vi "固定站CODMn测量流程.vi"(11 "控制命令":T1(ring)) -> ()   [LabVIEW 2016, in "斯坦道CODMn.lvlib"]
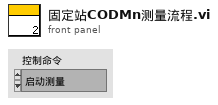
[diagram p1: front panel]
types:
  T1 = enum16{"启动测量", "标样核查", "零点核查", "跨度核查", "空白测试", "平行样测试", "加标回收", "空白校准", "标样校准", "初始化（清洗）", "停止测试", "仪器重启", "校时", "模式设置", "测量间隔设置"}
  T2 = cluster{"命令":string, "测量模式":enum16{"水样测量", "标样核查", "零点核查", "跨度核查", "空白测试", "加标回收", "平行样", "校零", "校标"}, "CODMn量程切换":enum32{"H", "L", "AUTO"}}
  T3 = cluster{"仪器":enum16{"", "氨氮", "总磷", "总氮", "CODMn", "CODCr"}, "启动命令":enum16{"启动水样流程", "启动加标流程", "排液", "停止", "柱塞泵启动"}}
  T4 = cluster{"时间标识":timestamp, "参数":string, "日志信息":string, "流程参数":string}
  T5 = enum16{"水样测量", "标样核查", "零点核查", "跨度核查", "空白测试", "加标回收", "平行样", "校零", "校标"}
  T6 = cluster{"时间标识":timestamp, "设备":string, "日志信息":string, "流程参数":string}
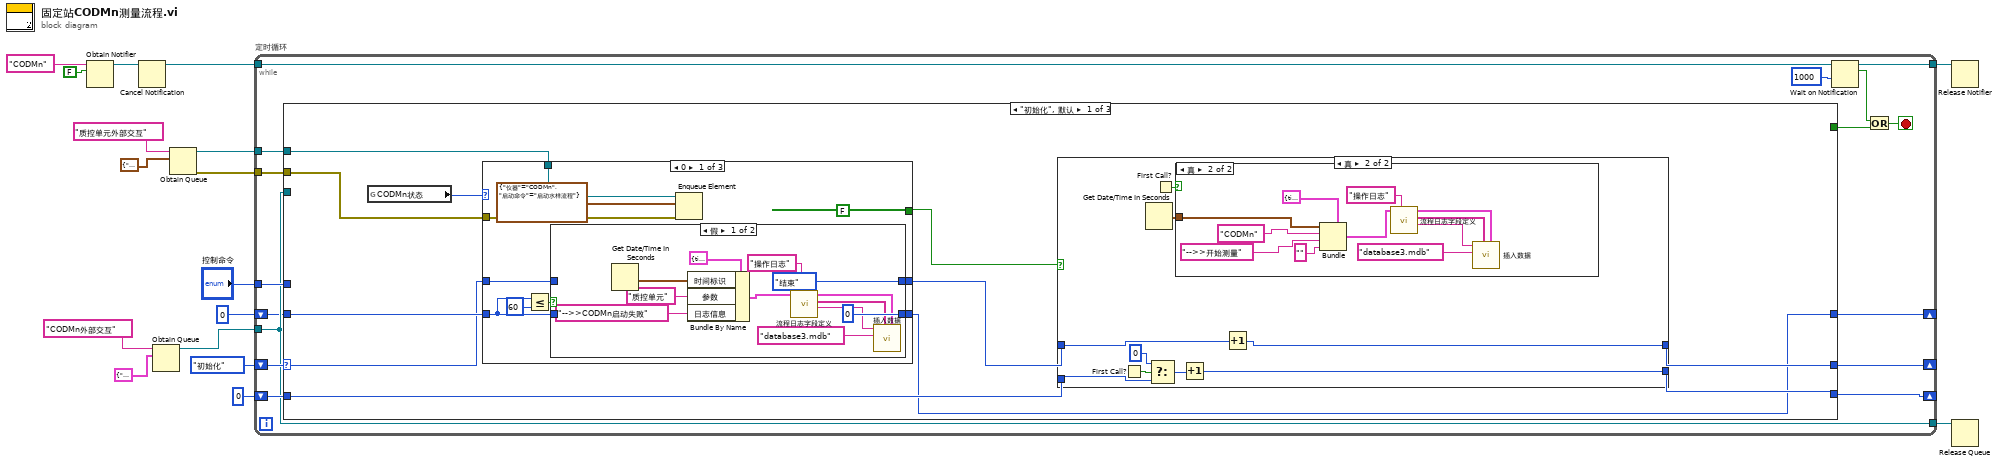
[diagram p0: block diagram]
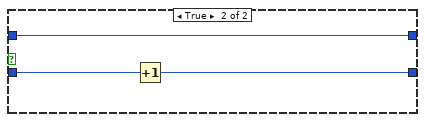
[diagram p4: hidden frame]
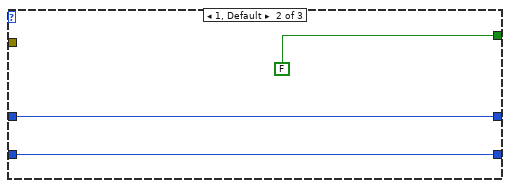
[diagram p5: hidden frame]
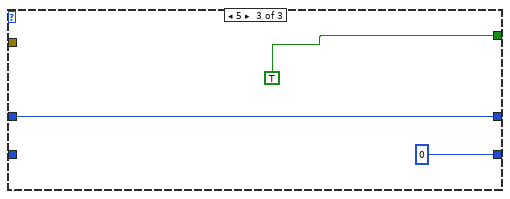
[diagram p6: hidden frame]
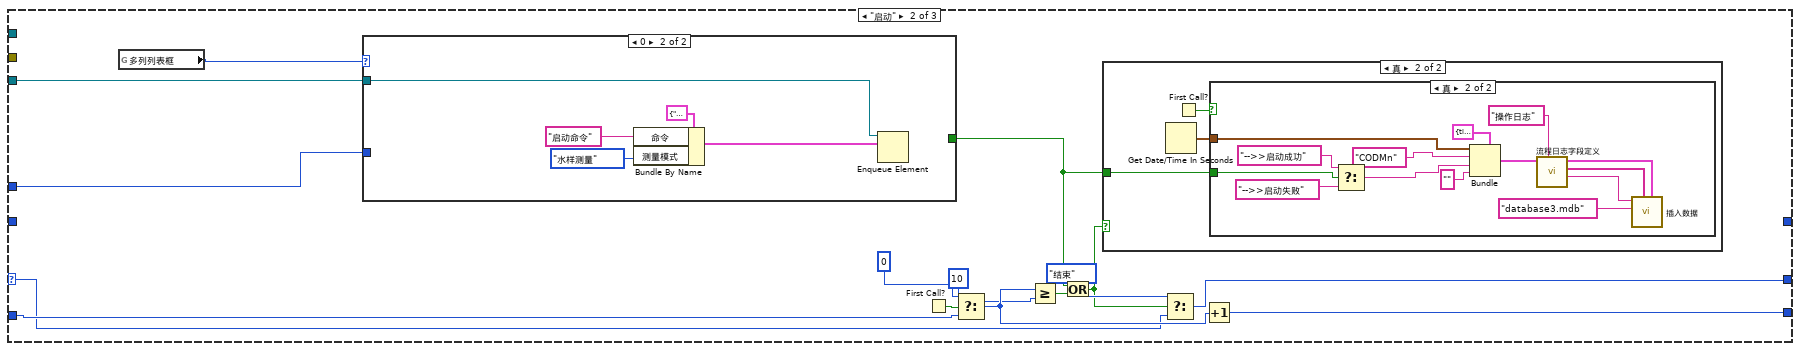
[diagram p7: hidden frame]
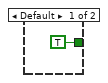
[diagram p10: hidden frame]
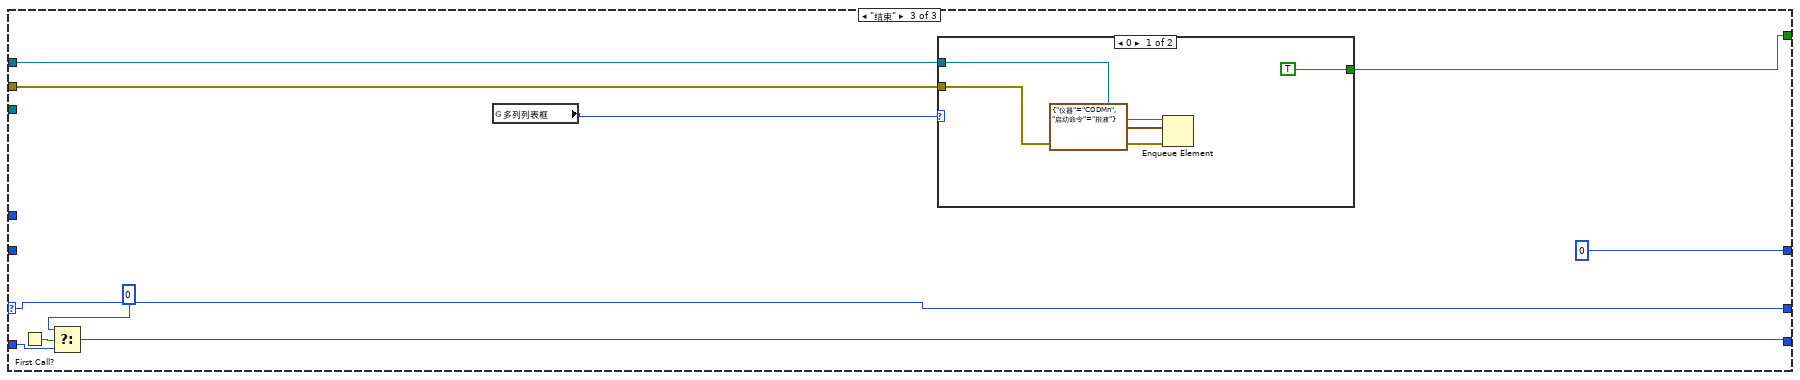
[diagram p11: hidden frame]
diagram:
  n1 = Obtain Notifier(name (unnamed)="CODMn" ("名称（未命名）"), notification data type=FALSE) -> (notifier out=w15:refnum<notifier>)  [unwired: 2 in, 2 out]
  n2 = Cancel Notification(0:w15) -> (8:w14:refnum<notifier>)  [unwired: 1 in, 2 out]
  n3 = Obtain Queue(name (unnamed)="CODMn外部交互" ("名称（未命名）"), element data type=T2 {"命令"="启动命令", "测量模式"=enum."水样测量", "CODMn量程切换"=enum."AUTO"} ("元素")) -> (queue out=w1:refnum<queue>)  [unwired: 3 in, 2 out]
  n4 = Obtain Queue(name (unnamed)="质控单元外部交互" ("名称（未命名）"), element data type=T3 {"仪器"=enum."氨氮", "启动命令"=enum."启动水样流程"} ("元素")) -> (queue out=w6:refnum<queue>, error out=w5:errorcluster)  [unwired: 3 in, 1 out]
  n5 = while "定时循环" {
    tunnel: w1 -> [w22]
    tunnel: w14 -> [w33]
    tunnel: "控制命令" -> [w28]
    shift-right: [w27] -> _
    shift-left: enum16{"初始化", "启动", "结束"}."初始化" -> [w29]
    shift-right: [w25] -> _
    shift-left: 0 -> [w26]
    tunnel: [w23] -> w10
    tunnel: [w22] -> w11
    tunnel: w6 -> [w21]
    tunnel: w5 -> [w20]
    shift-right: [w18] -> _
    shift-left: 0 -> [w19]
    stop <- w30 stop-if-true
    n6 = case shown="\"初始化\", 默认" w29 {
      selector: w29 -> [w36 w103 w145]
      tunnel: w28 -> [_ w112 _]
      tunnel: w22 -> [_ w111 _]
      tunnel: [w44 w104 w145] -> w27
      tunnel: w26 -> [w43 w108 w142]
      tunnel: [w42 w107 w141] -> w25
      tunnel: [_ _ w138] -> w24
      tunnel: w21 -> [w40 _ w140]
      tunnel: w20 -> [w39 _ w139]
      tunnel: w19 -> [w38 _ _]
      tunnel: [w37 _ 0] -> w18
      frame "初始化", Default {
        n7 = global read "CODMN外部API.vi" "CODMn状态"() -> (w34:u16)
        n8 = case shown="0" w34 {
          tunnel: [FALSE ("s") FALSE ("s") TRUE ("s")] -> w41
          tunnel: w40 -> [w75 _ _]
          tunnel: w39 -> [w74 _ _]
          tunnel: w38 -> [w72 w92 _]
          tunnel: [w69 w92 0] -> w37
          tunnel: w36 -> [w68 w93 w96]
          tunnel: [w67 w93 w96] -> w35
          frame 0 {
            n9 = Less Or Equal?(x=w72, y=60) -> (x <= y?=w70:bool)
            n10 = case shown="假" w70 {
              tunnel: w72 -> [_ w91]
              tunnel: [0 w90] -> w69
              tunnel: w68 -> [_ w89]
              tunnel: [enum16{"初始化", "启动", "结束"}."结束" w89] -> w67
              frame False {
                n11 = Get Date/Time In Seconds() -> (seconds since 1Jan1904=w84:timestamp)
                n12 = Bundle By Name(cluster=T4 {"时间标识"=timestamp(0 s since 1904-01-01), "参数"="", "日志信息"="", "流程参数"=""} ("data in"), "时间标识"=w84, "参数"="质控单元" ("设备"), "日志信息"="-->>CODMn启动失败") -> (w78:T4)
                n13 = call "流程日志字段定义.vi"("table输入"="操作日志", "data in"=w78) -> ("table输出"=w81:string, "columns"=w82:string[], "data out"=w83:T6)  [unwired: 7 in]
                n14 = call "插入数据.vi"("data"=w83, "columns"=w82, "database"="database3.mdb", "table"=w81) -> ()  [unwired: 7 in, 1 out]
              }
              frame True {
                n15 = Increment(x=w91) -> (x+1=w90:i32)
              }
            }
            n16 = Enqueue Element(queue=w75, element=T3 {"仪器"=enum."CODMn", "启动命令"=enum."启动水样流程"} ("元素"), error in (no error)=w74) -> ()  [unwired: 1 in, 3 out]
          }
          frame 1, Default {
          }
          frame 5 {
          }
        }
        n17 = case shown="真" w41 {
          tunnel: w35 -> [w46 w53]
          tunnel: [w46 w52] -> w44
          tunnel: w43 -> [w45 w50]
          tunnel: [w45 w47] -> w42
          frame False {
          }
          frame True {
            n18 = First Call?() -> (First Call?: T/F=w51:bool)
            n19 = Get Date/Time In Seconds() -> (seconds since 1Jan1904=w55:timestamp)
            n20 = Select(t=0, s=w51, f=w50) -> (s? t:f=w48:i32)
            n21 = First Call?() -> (First Call?: T/F=w54:bool)
            n22 = case shown="真" w54 {
              tunnel: w55 -> [_ w63]
              frame False {
              }
              frame True {
                n23 = Bundle(cluster=T4 {"时间标识"=timestamp(0 s since 1904-01-01), "参数"="", "日志信息"="", "流程参数"=""} ("data in"), "时间标识"=w63, "参数"="CODMn" ("设备"), "日志信息"="-->>开始测量", "流程参数"="" ("table输入")) -> (w56:T4)
                n24 = call "流程日志字段定义.vi"("table输入"="操作日志", "data in"=w56) -> ("table输出"=w59:string, "columns"=w58:string[], "data out"=w57:T6)  [unwired: 7 in]
                n25 = call "插入数据.vi"("data"=w57, "columns"=w58, "database"="database3.mdb", "table"=w59) -> ()  [unwired: 7 in, 1 out]
              }
            }
            n26 = Increment(x=w48) -> (x+1=w47:i32)
            n27 = Increment(x=w53) -> (x+1=w52:enum16{"初始化", "启动", "结束"})
          }
        }
      }
      frame "启动" {
        n28 = global read "运行时序全局变量.vi" "多列列表框"() -> (w98:i32)
        n29 = case shown="0" w98 {
          tunnel: w112 -> [_ _]
          tunnel: w111 -> [_ w135]
          tunnel: [TRUE _] -> w99
          frame Default {
          }
          frame 0 {
            n30 = Bundle By Name(cluster=T2 {"命令"="启动命令", "测量模式"=enum."水样测量", "CODMn量程切换"=enum."AUTO"} ("元素"), "命令"="启动命令", "测量模式"=T5."水样测量") -> (w132:T2)
            n31 = Enqueue Element(queue=w135, element=w132) -> ()  [unwired: 2 in, 3 out]
          }
        }
        n32 = First Call?() -> (First Call?: T/F=w110:bool)
        n33 = Select(t=0, s=w110, f=w108) -> (s? t:f=w106:i32)
        n34 = Greater Or Equal?(x=w106, y=10) -> (x >= y?=w102:bool)
        n35 = Or(x=w99, y=w102) -> (x .or. y?=w100:bool)
        n36 = case shown="真" w100 {
          tunnel: w99 -> [_ w113]
          frame False {
          }
          frame True {
            n37 = Get Date/Time In Seconds() -> (seconds since 1Jan1904=w114:timestamp)
            n38 = First Call?() -> (First Call?: T/F=w115:bool)
            n39 = case shown="真" w115 {
              tunnel: w114 -> [_ w118]
              tunnel: w113 -> [_ w129]
              frame False {
              }
              frame True {
                n40 = Select(t="-->>启动成功" ("日志信息"), s=w129, f="-->>启动失败" ("日志信息")) -> (s? t:f=w116:string)
                n41 = Bundle(cluster=T4 {"时间标识"=timestamp(0 s since 1904-01-01), "参数"="", "日志信息"="", "流程参数"=""} ("data in"), "时间标识"=w118, "参数"="CODMn" ("设备"), "日志信息"=w116, "流程参数"="" ("table输入")) -> (w124:T4)
                n42 = call "流程日志字段定义.vi"("table输入"="操作日志", "data in"=w124) -> ("table输出"=w121:string, "columns"=w120:string[], "data out"=w119:T6)  [unwired: 7 in]
                n43 = call "插入数据.vi"("data"=w119, "columns"=w120, "database"="database3.mdb", "table"=w121) -> ()  [unwired: 7 in, 1 out]
              }
            }
          }
        }
        n44 = Select(t=enum16{"初始化", "启动", "结束"}."结束", s=w100, f=w103) -> (s? t:f=w104:enum16{"初始化", "启动", "结束"})
        n45 = Increment(x=w106) -> (x+1=w107:i32)
      }
      frame "结束" {
        n46 = First Call?() -> (First Call?: T/F=w144:bool)
        n47 = Select(t=0, s=w144, f=w142) -> (s? t:f=w141:i32)
        n48 = global read "运行时序全局变量.vi" "多列列表框"() -> (w136:i32)
        n49 = case shown="0" w136 {
          tunnel: w140 -> [w148 _]
          tunnel: w139 -> [w147 _]
          tunnel: [TRUE _] -> w138
          frame 0 {
            n50 = Enqueue Element(queue=w148, element=T3 {"仪器"=enum."CODMn", "启动命令"=enum."排液"} ("元素"), error in (no error)=w147) -> ()  [unwired: 1 in, 3 out]
          }
          frame 1, Default {
          }
        }
      }
    }
    n51 = Wait on Notification(notifier=w33, timeout in ms (-1)=1000 ("超时毫秒(-1)")) -> (notifier out=w23:refnum<notifier>, notification=w31:bool)  [unwired: 2 in, 2 out]
    n52 = Or(x=w31, y=w24) -> (x .or. y?=w30:bool)
  }
  n53 = Release Notifier(notifier=w10) -> ()  [unwired: 2 in, 3 out]
  n54 = Release Queue(queue=w11) -> ()  [unwired: 2 in, 3 out]
